vi "Write Expected resulting path.vi"(8 "error in (no error)":errorcluster, 10 "Expected resulting path":string, 11 "[Test Case] Build path in":refnum<class "[Test Case] Build path.lvclass">) -> (0 "error out":errorcluster, 3 "[Test Case] Build path out":refnum<class "[Test Case] Build path.lvclass">)   [LabVIEW 2015, in "Tests.lvlib" / "[Test Case] Build path.lvclass"]
uses:
  [Test Case] Build path.lvclass
  [Test Case] Build path.lvclass/[Test Case] Build path.ctl
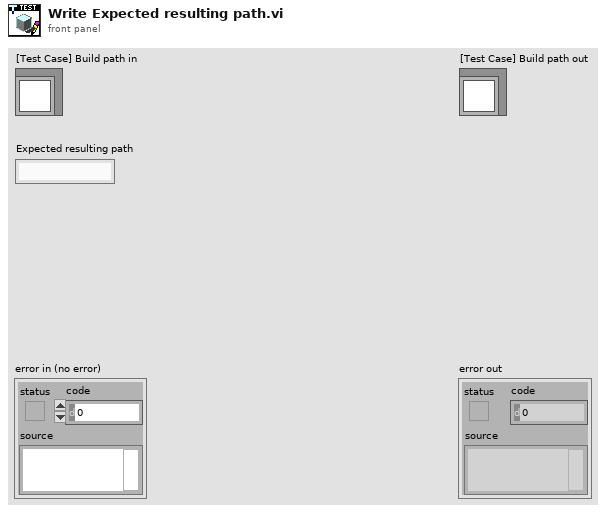
[diagram p1: front panel]
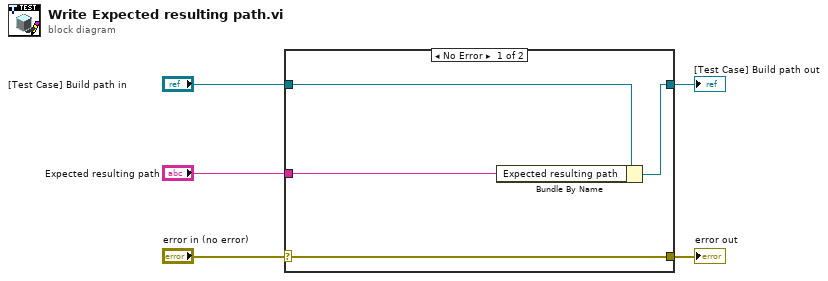
[diagram p0: block diagram]
diagram:
  n1 = case shown="No Error" "error in (no error)" {
    selector: "error in (no error)" -> [w9 w10]
    tunnel: [w9 w10] -> w4
    tunnel: [w7 w11] -> w2
    tunnel: "[Test Case] Build path in" -> [w8 w11]
    tunnel: "Expected resulting path" -> [w6 _]
    frame No Error {
      n2 = Bundle By Name(cluster=w8, "Expected resulting path"=w6) -> (w7:refnum<class "[Test Case] Build path.lvclass">)
    }
    frame Error {
    }
  }
  "error out" <- w4
  "[Test Case] Build path out" <- w2
